vi "搜索所有匹配元素(2D Path).vi"(8 "error in (no error)":errorcluster caption="错误输入（无错误）", 9 "开始索引（0）":i32, 10 "元素":path, 11 "数组":path[][](array[path])) -> (0 "error out":errorcluster caption="错误输出", 1 "匹配数量":i32, 3 "匹配元素索引":cluster{"行":i32, "列":i32}[](array[cluster]))   [LabVIEW 2012]
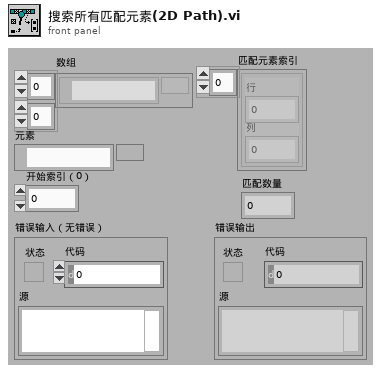
[diagram p1: front panel]
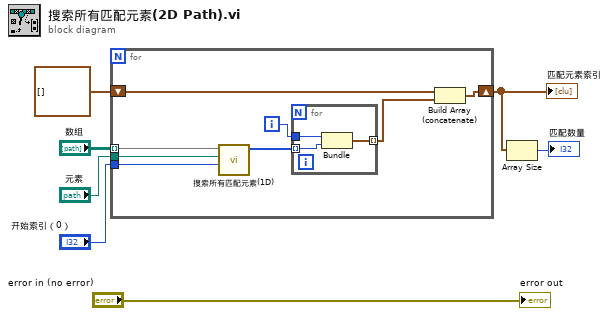
[diagram p0: block diagram]
diagram:
  n1 = for {
    tunnel: "数组" -> [w15] mode=indexing
    tunnel: "元素" -> [w14]
    tunnel: "开始索引（0）" -> [w13]
    shift-right: [w8] -> w2
    shift-left: cluster{i32, "数值":i32}[] [] -> [w10]
    i -> [w11]
    n2 = call-poly "搜索所有匹配元素(1D).vi"("开始索引（0）"=w13, "元素"=w14, "数组"=w15) -> ("匹配元素索引"=w12:i32[])  [unwired: 6 in, 2 out]
    n3 = for {
      tunnel: w12 -> [w18] mode=indexing
      tunnel: w11 -> [w17]
      tunnel: [w16] -> w9 mode=indexing
      n4 = Bundle(w17, "数值"=w18) -> (w16:cluster{i32, "数值":i32})  [unwired: 1 in]
    }
    n5 = Build Array (concatenate)(w10, w9) -> (w8:cluster{i32, "数值":i32}[])
  }
  "匹配元素索引" <- w2
  n6 = Array Size(array=w2) -> (size(s)=→"匹配数量":i32)
  "error out" <- "error in (no error)"
